vi "JJMCclase7 trabajo.vi"() -> ()   [LabVIEW 2013]
panel:
  out "suma 150":dbl
  out "contador":dbl
  out "promedio":dbl
  out "velocidad":dbl(knob) scale=0.0..220.0
  # "generar 10 pruebas de velocidad luego sumar las velocidades mayores a 150 y obtener su promedio"
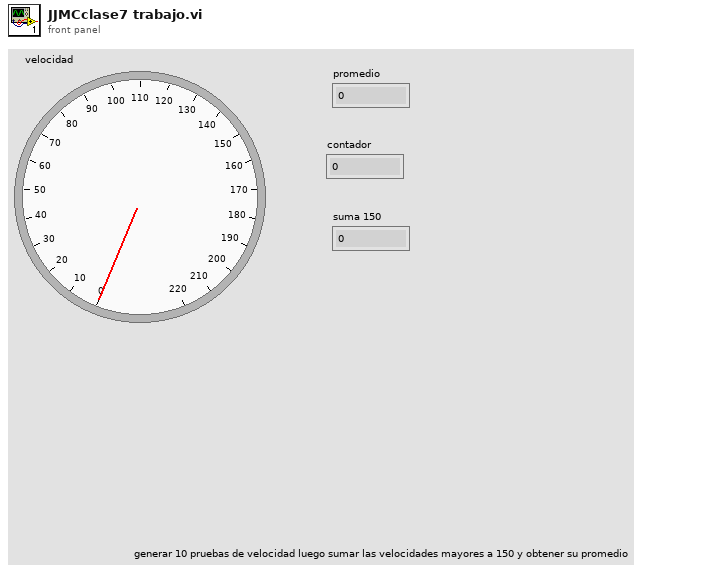
[diagram p1: front panel]
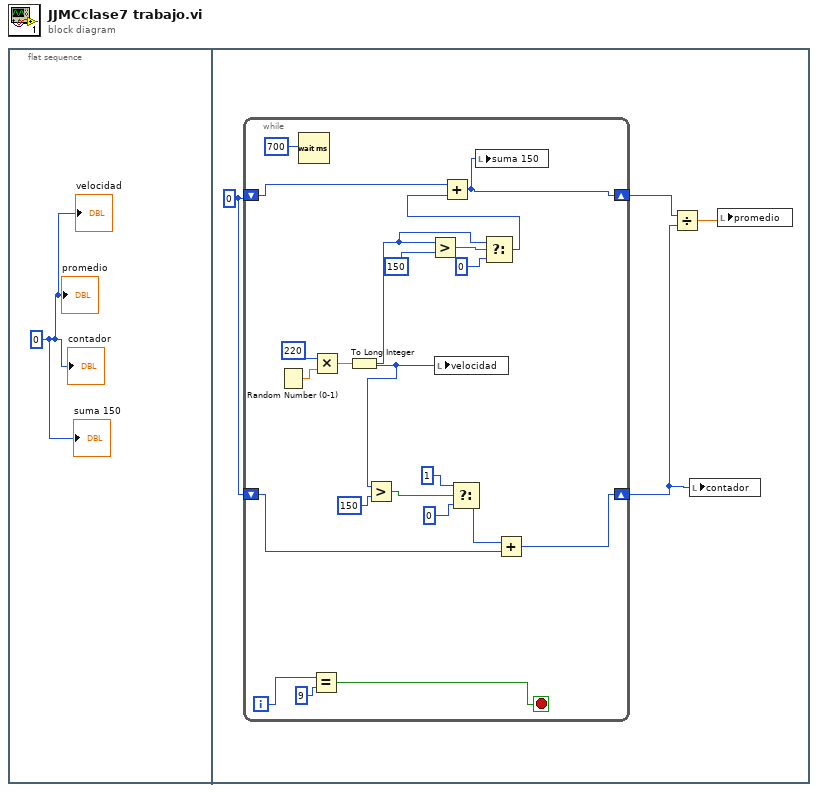
[diagram p0: block diagram]
diagram:
  n1 = flat-sequence {
    frame #0 {
      w1 = 0
      "velocidad" <- w1
      "promedio" <- w1
      "contador" <- w1
      "suma 150" <- w1
    }
    frame #1 {
      w3 = 0
      n2 = while {
        shift-right: [w12] -> w5
        shift-left: w3 -> [w26]
        shift-right: [w6] -> w2
        shift-left: w3 -> [w9]
        i -> [w17]
        stop <- w16 stop-if-true
        n3 = Random Number (0-1)() -> (number: 0 to 1=w24:dbl)
        n4 = Wait (ms)(milliseconds to wait=700) -> ()  [unwired: 1 out]
        n5 = Equal?(x=w17, y=9) -> (x = y?=w16:bool)
        n6 = Multiply(x=220, y=w24) -> (x*y=w23:dbl)
        n7 = To Long Integer(number=w23) -> (32bit integer=w10:i32)
        n8 = Greater?(x=w10, y=150) -> (0:w14:bool)
        n9 = Greater?(x=w10, y=150) -> (0:w21:bool)
        n10 = local write "velocidad"(w10) -> ()
        n11 = Select(t=1, s=w14, f=0) -> (s? t:f=w7:i32)
        n12 = Select(t=w10, s=w21, f=0) -> (s? t:f=w19:i32)
        n13 = Add(x=w26, y=w19) -> (x+y=w12:i32)
        n14 = local write "suma 150"(w12) -> ()
        n15 = Add(x=w7, y=w9) -> (x+y=w6:i32)
      }
      n16 = Divide(x=w5, y=w2) -> (x/y=w4:dbl)
      n17 = local write "contador"(w2) -> ()
      n18 = local write "promedio"(w4) -> ()
    }
  }
